vi "PH_Beckhoff_StepMot.Set BaseClass Changes to Beckhoff Configuration.vi"(0 "i ref in":refnum<vi>, 5 "error in":errorcluster) -> (14 "i ref out":refnum<vi>, 16 "Config changed?":bool, 19 "error out":errorcluster)   [LabVIEW 2014, in "PH_Beckhoff_StepMot.lvlib"]
doc: "This VI checks whether base class conditions have been changed which makes it necessary to reconfigure the 6P."
uses:
  PH_Beckhoff_StepMot.lvlib
  PH_Beckhoff_StepMot.Axis Cluster.ctl
  non_GPL/instr.lib/Beckhoff/Specials/Step Motor Klemmen/Beckhoff.Step Motor - Motor Configuration.ctl
  non_GPL/instr.lib/Beckhoff/Read and Write Register/Step Motor Klemmen/Beckhoff.Step Motor - Feature Register 1.ctl
  non_GPL/instr.lib/Beckhoff/Read and Write Register/Step Motor Klemmen/Beckhoff.Step Motor - Feature Register 2.ctl
  PH_Stepmotor_BaseClass/PH_Stepmotor_BaseClass.lvlib
  non_GPL/instr.lib/Beckhoff/Beckhoff - Driver np.lvlib
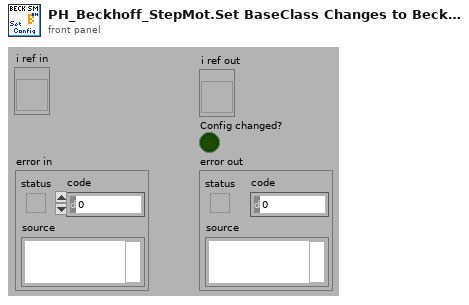
[diagram p1: front panel]
types:
  T1 = typedef "PH_Stepmotor_BaseClass.lvlib/PH_Stepmotor_BaseClass.i attribute.ctl" = cluster{"Device Error":errorcluster, "Axes PSDB Thread":cluster{"Ref":refnum<vi>, "Q-Ref":refnum<queue>, "Data Status":T2}, "Axes":T3[], "Axes PSDB Infos":cluster{"GUI Name":string, "PSDB Instance ID":i32, "PSDB Status Service ID":i32, "Axis":i32, "Class":string}[], "GUI Refs":T8}
  T2 = typedef "PH_PSDBWriter.lvlib/PH_PSDBWriter.Data Status.ctl" = i16
  T3 = typedef "PH_Stepmotor_BaseClass.lvlib/PH_Stepmotor_BaseClass.Axis Attributes.ctl" = cluster{"Settings":T4, "Endswitch?":bool, "DIM Service IDs":T6, "Activity":T7, "Configured?":bool, "Position":cluster{"Current":i32, "Target":i32}, "Position to set":cluster{"New?":bool, "Wanted":i32}, "Stop?":bool, "Reset?":bool, "Move?":bool, "Nothing connected?":bool}
  T4 = typedef "PH_Stepmotor_BaseClass.lvlib/PH_Stepmotor_BaseClass.Axis Settings.ctl" = cluster{"Sign change":bool, "Width":dbl, "Calibration":dbl, "Unit":string, "Motor Type":T5, "Unit Width":string, "Unit CF":string}
  T5 = typedef "PH_Stepmotor_BaseClass.lvlib/PH_Stepmotor_BaseClass.Motor Type.ctl" = enum16{"Unspecific", "OWIS 49.120.2633", "OWIS 49.060.1033", "OWIS 43.040.2558", "Diamond Motion 2200 series", "OWIS 49.120.266B.MV6", "Calorimeter", "Linear Stage 1", "MICOS VT-80", "MICOS VT-80 S", "Standa Rotstage nt0.95A", "PUF RA 320.200", "PUF RA 800.200", "PUF RA 800.400", "PUF RA 400.50", "1324.nn.800.50", "1324.n9c.800.50", "1324.nn.320.200", "1324.nn.400.200", "1324.nn.800.200", "1324.nn.400.50", "1324.8c9c.800.50", "1324.8c9c.400.200"}
  T6 = typedef "PH_Stepmotor_BaseClass.lvlib/PH_Stepmotor_BaseClass.Axis DIM Service IDs.ctl" = cluster{"Settings":i32, "Information":i32}
  T7 = typedef "PH_Stepmotor_BaseClass.lvlib/PH_Stepmotor_BaseClass.Axis Activity.ctl" = enum16{"No Information", "stopped", "running", "Failure", "Alarm", "stopped at backward ES", "stopped at foreward ES"}
  T8 = typedef "PH_Stepmotor_BaseClass.lvlib/PH_Stepmotor_BaseClass.GUI Refs.ctl" = cluster{"Axes Configuration":refnum<vi>, "Device Error":refnum<vi>, "Axes PSDB Infos":refnum<vi>}
  T9 = typedef "PH_Beckhoff_StepMot.lvlib/PH_Beckhoff_StepMot.Axis Cluster.ctl" = cluster{"Step Motor Configuration":T10, "To set?":bool, "Endswitch inverted?":bool}
  T10 = typedef "Beckhoff - Driver np.lvlib/Beckhoff.Step Motor - Motor Configuration.ctl" = cluster{"Feature Register":T11, "I max A [mA]":dbl, "I max B [mA]":dbl, "v min":u32, "v max":u32, "a max":u32, "I hold [%]":u32, "Steps/qp":u32, "Feature Register 2":T12}
  T11 = typedef "Beckhoff - Driver np.lvlib/Beckhoff.Step Motor - Feature Register 1.ctl" = cluster{"en Auto Start":bool, "en Auto Stop":bool, "dis Wd Timer":bool, "OP Mode 1":bool, "OP Mode 2":bool, "Ramp Type":bool, "inv Pos Feedback":bool, "en User Cur Table":bool, "en Latch Evt Clr Pos":bool, "en Multi Latch Vals":bool, "en Sign Disp*":bool, "Feedback Type*":bool, "en neg Gate Lock*":bool, "en pos Gate Lock*":bool, "dis Enc Fltr*":bool, "en Counter Mode*":bool}
  T12 = typedef "Beckhoff - Driver np.lvlib/Beckhoff.Step Motor - Feature Register 2.ctl" = cluster{"rev Homing Dir":bool, "en Decac Ramp":bool, "Latch Reg Pos":bool, "Show Idle":bool, "dis Ref Input 1":bool, "dis Ref Input 2":bool, "en ext Auto Start":bool, "N/A":bool, "N/A":bool, "N/A":bool, "N/A":bool, "N/A":bool, "en Clr Proc Data":bool, "en Man Ecl Tolerce*":bool, "rev Dig Input 1":bool, "rev Dig Input 2":bool}
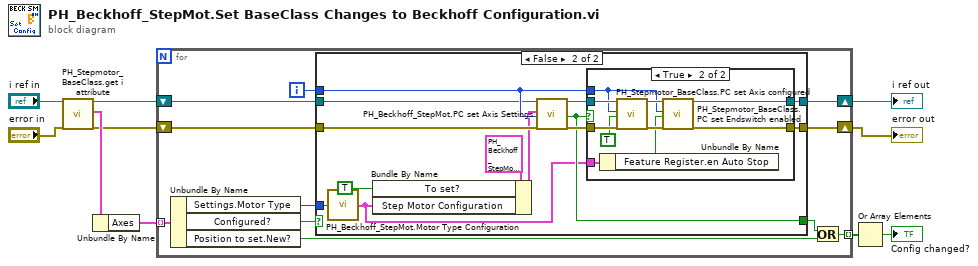
[diagram p0: block diagram]
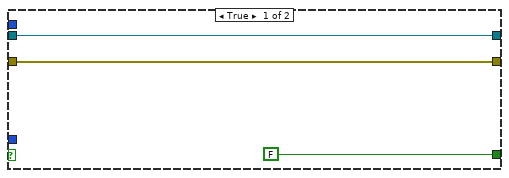
[diagram p2: hidden frame]
diagram:
  n1 = call "PH_Stepmotor_BaseClass.get i attribute.vi"("i ref in"="i ref in", "error in (no error)"="error in") -> ("i ref out"=w2:refnum<vi>, "i attribute"=w8:T1, "error out"=w1:errorcluster)  [unwired: 15 in]
  n2 = Unbundle By Name(w8) -> ("Axes"=w3:T3[])
  n3 = for {
    shift-right: [w17] -> w5
    shift-left: w1 -> [w21]
    shift-right: [w16] -> w6
    shift-left: w2 -> [w18]
    tunnel: w3 -> [w20] mode=indexing
    tunnel: [w14] -> w7 mode=indexing
    i -> [w15]
    n4 = Unbundle By Name(w20) -> ("Settings.Motor Type"=w19:T5, "Configured?"=w11:bool, "Position to set.New?"=w13:bool)
    n5 = case shown="False" w11 {
      tunnel: w21 -> [w23 w32]
      tunnel: w19 -> [_ w37]
      tunnel: w18 -> [w24 w33]
      tunnel: [w23 w36] -> w17
      tunnel: [w24 w35] -> w16
      tunnel: w15 -> [_ w34]
      tunnel: [FALSE w26] -> w12
      frame True {
      }
      frame False {
        n6 = call "PH_Beckhoff_StepMot.Motor Type Configuration.vi"("Motor Type"=w37) -> ("Step Motor Configuration"=w25:T10)
        n7 = Bundle By Name(cluster=T9 {"Step Motor Configuration"={"Feature Register"={"en Auto Start"=FALSE, "en Auto Stop"=FALSE, "dis Wd Timer"=FALSE, "OP Mode 1"=FALSE, "OP Mode 2"=FALSE, "Ramp Type"=FALSE, "inv Pos Feedback"=FALSE, "en User Cur Table"=FALSE, "en Latch Evt Clr Pos"=FALSE, "en Multi Latch Vals"=FALSE, "en Sign Disp*"=FALSE, "Feedback Type*"=FALSE, "en neg Gate Lock*"=FALSE, "en pos Gate Lock*"=FALSE, "dis Enc Fltr*"=FALSE, "en Counter Mode*"=FALSE}, "I max A [mA]"=0.0, "I max B [mA]"=0.0, "v min"=0, "v max"=0, "a max"=0, "I hold [%]"=0, "Steps/qp"=0, "Feature Register 2"={"rev Homing Dir"=FALSE, "en Decac Ramp"=FALSE, "Latch Reg Pos"=FALSE, "Show Idle"=FALSE, "dis Ref Input 1"=FALSE, "dis Ref Input 2"=FALSE, "en ext Auto Start"=FALSE, "N/A"=FALSE, "N/A"=FALSE, "N/A"=FALSE, "N/A"=FALSE, "N/A"=FALSE, "en Clr Proc Data"=FALSE, "en Man Ecl Tolerce*"=FALSE, "rev Dig Input 1"=FALSE, "rev Dig Input 2"=FALSE}}, "To set?"=FALSE, "Endswitch inverted?"=FALSE} ("Axis Settings"), "To set?"=TRUE, "Step Motor Configuration"=w25) -> (w30:T9)
        n8 = call "PH_Beckhoff_StepMot.PC set Axis Settings.vi"("VI in"=w33, "Axis Settings"=w30, "Axis"=w34, "error in (no error)"=w32) -> ("VI out"=w28:refnum<vi>, "Settings changed?"=w26:bool, "error out"=w27:errorcluster)  [unwired: 13 in]
        n9 = case shown="True" w26 {
          tunnel: w27 -> [w38 w49]
          tunnel: [w38 w43] -> w36
          tunnel: w28 -> [w39 w48]
          tunnel: [w39 w45] -> w35
          tunnel: w34 -> [_ w42]
          tunnel: w25 -> [_ w41]
          frame False {
          }
          frame True {
            n10 = Unbundle By Name(w41) -> ("Feature Register.en Auto Stop"=w40:bool)
            n11 = call "PH_Stepmotor_BaseClass.PC set Axis configured.vi"("VI in"=w48, "Axis"=w42, "Configured?"=TRUE, "error in (no error)"=w49) -> ("VI out"=w46:refnum<vi>, "error out"=w44:errorcluster)  [unwired: 14 in]
            n12 = call "PH_Stepmotor_BaseClass.PC set Endswitch enabled.vi"("VI in"=w46, "axis"=w42, "Endswitch?"=w40, "error in (no error)"=w44) -> ("VI out"=w45:refnum<vi>, "error out"=w43:errorcluster)  [unwired: 14 in]
          }
        }
      }
    }
    n13 = Or(x=w12, y=w13) -> (x .or. y?=w14:bool)
  }
  "i ref out" <- w6
  "error out" <- w5
  n14 = Or Array Elements(Boolean array=w7) -> (logical OR=→"Config changed?":bool)
